vi "Swerve_Module Drive Config.vi"(5 "Max # Of Tries":i32, 6 "Send Cmd Timout(ms)":u32=300, 7 "Module Specific Data":T1, 8 "Error":errorcluster, 9 "Module Drive Config Data":T8={"ModuleDrive Ver"=0, "Output"={"Type"=enum."Counter-Clockwise", "Neutral"=enum."EEPROMSetting", "Max"={"FWD"=0.0, "REV"=0.0}, "Min"={"FWD"=0.0, "REV"=0.0}, "OL Ramp Rate (S)"=0.0, "Dead Band"=0.0}, "CL"={"Gains"={"P"=1.0, "I"=0.01, "D"=0.0, "F"=0.0}, "Error Allowed"={"High"=0.0, "Low"=0.0}, "I Zone"={"High"=10000.0, "Low"=-1000.0}, "Max Out"={"FWD"=1.0, "REV"=-1.0}, "Max I Accu"={"High"=10.0, "Low"=-10.0}, "CL Ramp Rate (S)"=0.0}, "VoltageComp"={"Enable"=FALSE, "Value"=0.0}} {"Output"."Min"."REV" format="%.2f"; "Output"."Min"."FWD" format="%.2f"; "Output"."Max"."REV" format="%.2f"; "Output"."Max"."FWD" format="%.2f"; "VoltageComp"."Value" format="%.1g"; "CL"."Max I Accu"."Low" format="%#.8f"; "CL"."Max I Accu"."High" format="%#.8f"; "CL"."Gains"."F" format="%#.8f"; "CL"."Gains"."D" format="%#.8f"; "CL"."Gains"."I" format="%#.8f"; "CL"."Gains"."P" format="%#.8f"; "CL"."Error Allowed"."Low" format="%#.8f"; "CL"."Error Allowed"."High" format="%#.8f"; "CL"."I Zone"."Low" format="%#.8f"; "CL"."I Zone"."High" format="%#.8f"; "CL"."Max Out"."REV" format="%.2f"; "CL"."Max Out"."FWD" format="%.2f"}, 11 "PhoenixMotorControlDevRef":T3={"DeviceStatus"={"status"=FALSE, "code"=0, "source"=""}, "Type"=enum."PWM", "PWM"={"PWM Channel"=enum."Invalid", "DeadBand"={"Name"="", "maxPositivePwm"=0, "minPositivePwm"=0, "centerPwm"=0, "maxNegativePwm"=0, "minNegativePwm"=0, "angularRange"=0}}, "CAN"={"Device Number"=0, "SetOutput VI Ref"=variant, "GetOutput VI Ref"=variant, "Enable VI Ref"=variant, "Disable VI Ref"=variant, "Data"=variant}, "Invert"=FALSE, "DIO PWM"={"PWM \"Enable\" Channel"=enum."Invalid", "DIOChannel"=enum."Invalid", "PWM Rate"=0.0}}) -> (0 "Error Out":errorcluster, 3 "PhoenixMotorControlDevRef Out Out":T3)   [LabVIEW 2023]
uses:
  <vilib>/Utility/Data Type/NI_Data Type.lvlib
  <vilib>/Rock Robotics/WPI/ThirdParty/Phoenix-LabVIEW/Motor Controller/Controls/CTRE_Phoenix_MotorControl_NeutralMode.ctl
  <vilib>/Rock Robotics/SystemInterfaces/DIO/FPGA_DIOPWMChannel.ctl
  <vilib>/Rock Robotics/WPI/PWM/WPI_PWMDeadband.ctl
  <vilib>/Rock Robotics/WPI/MotorControl/WPI_MotorControlType.ctl
  <vilib>/Rock Robotics/SystemInterfaces/DIO/FPGA_DIOChannel.ctl
  <vilib>/Rock Robotics/WPI/MotorControl/WPI_MotorControlDeviceRef.ctl
  Shared Code/TypeDefs/Cluster_High-Low.ctl
  Shared Code/TypeDefs/Cluster_PID Gains.ctl
  Shared Code/TypeDefs/Cluster_PID Config.ctl
  <vilib>/Rock Robotics/WPI/ThirdParty/Phoenix-LabVIEW/Motor Controller/Controls/CTRE_Phoenix_MotorControl_TalonFXInvertType.ctl
  Shared Code/TypeDefs/Cluster_Enable-Value DBL.ctl
  Shared Code/TypeDefs/Cluster_Swerve Module Drive Config Data.ctl
  Shared Code/TypeDefs/ENUM_Motor Index.ctl
  Shared Code/TypeDefs/Cluster_Module Specific Config Data.ctl
  Shared Code/TypeDefs/Cluster_FWD  REV Values.ctl
  Shared Code/TypeDefs/Cluster_Config Motor Output.ctl
panel:
  # "Tune to Output\nto 1023 Max"
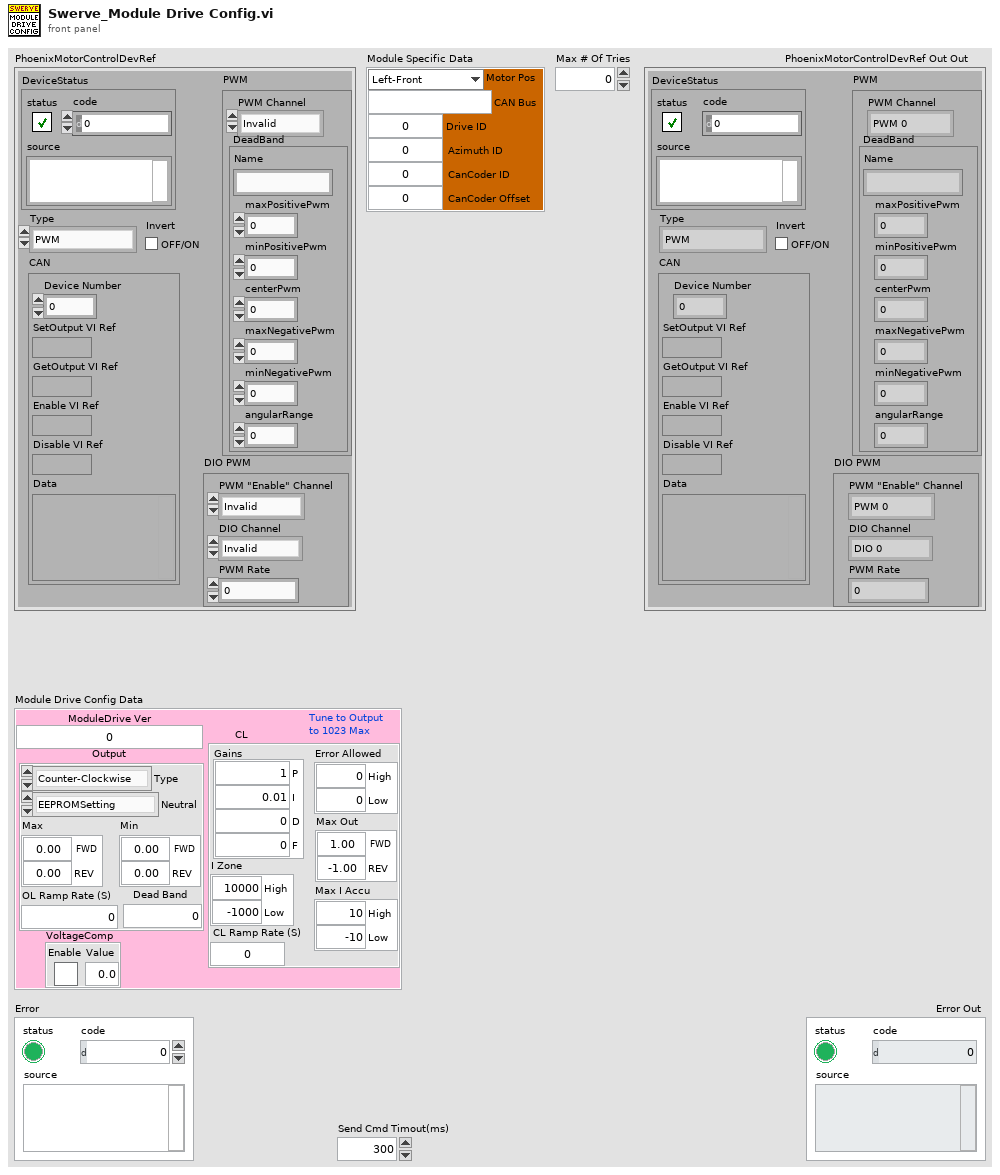
[diagram p1: front panel]
types:
  T1 = typedef "Cluster_Module Specific Config Data.ctl" = cluster{"Motor Pos":T2, "CAN Bus":string, "Drive ID":u8, "Azimuth ID":u8, "CanCoder ID":u8, "CanCoder Offset":dbl}
  T2 = typedef "ENUM_Motor Index.ctl" = enum16{"Left-Front", "Right-Front", "Left-Back", "Right-Back"}
  T3 = typedef "WPI_MotorControlDeviceRef.ctl" = cluster{"DeviceStatus":errorcluster, "Type":T4, "PWM":cluster{"PWM Channel":T5, "DeadBand":T6}, "CAN":cluster{"Device Number":u8, "SetOutput VI Ref":variant, "GetOutput VI Ref":variant, "Enable VI Ref":variant, "Disable VI Ref":variant, "Data":variant}, "Invert":bool, "DIO PWM":cluster{"PWM \"Enable\" Channel":T5, "DIOChannel":T7, "PWM Rate":dbl}}
  T4 = typedef "WPI_MotorControlType.ctl" = enum16{"PWM", "CAN", "DIO PWM"}
  T5 = typedef "FPGA_DIOPWMChannel.ctl" = enum8{"PWM 0", "PWM 1", "PWM 2", "PWM 3", "PWM 4", "PWM 5", "PWM 6", "PWM 7", "PWM 8", "PWM 9", "PWM MXP 0", "PWM MXP 1", "PWM MXP 2", "PWM MXP 3", "PWM MXP 4", "PWM MXP 5", "PWM MXP 6", "PWM MXP 7", "PWM MXP 8", "PWM MXP 9", "Invalid"}
  T6 = typedef "WPI_PWMDeadband.ctl" = cluster{"Name":string, "maxPositivePwm":i32, "minPositivePwm":i32, "centerPwm":i32, "maxNegativePwm":i32, "minNegativePwm":i32, "angularRange":u16}
  T7 = typedef "FPGA_DIOChannel.ctl" = enum8{"DIO 0", "DIO 1", "DIO 2", "DIO 3", "DIO 4", "DIO 5", "DIO 6", "DIO 7", "DIO 8", "DIO 9", "DIO MXP 0", "DIO MXP 1", "DIO MXP 2", "DIO MXP 3", "DIO MXP 4", "DIO MXP 5", "DIO MXP 6", "DIO MXP 7", "DIO MXP 8", "DIO MXP 9", "DIO MXP 10", "DIO MXP 11", "DIO MXP 12", "DIO MXP 13", "DIO MXP 14", "DIO MXP 15", "SPI Port CS1", "SPI Port CS2", "SPI Port CS3", "SPI Port MISO", "SPI Port MOSI", "Invalid"}
  T8 = typedef "Cluster_Swerve Module Drive Config Data.ctl" = cluster{"ModuleDrive Ver":u64, "Output":T9, "CL":T13, "VoltageComp":T16}
  T9 = typedef "Cluster_Config Motor Output.ctl" = cluster{"Type":T10, "Neutral":T11, "Max":T12, "Min":T12, "OL Ramp Rate (S)":dbl, "Dead Band":dbl}
  T10 = typedef "CTRE_Phoenix_MotorControl_TalonFXInvertType.ctl" = enum16{"Counter-Clockwise", "Clockwise"}
  T11 = typedef "CTRE_Phoenix_MotorControl_NeutralMode.ctl" = enum8{"EEPROMSetting", "Override to Coast", "Override to Brake"}
  T12 = typedef "Cluster_FWD  REV Values.ctl" = cluster{"FWD":dbl, "REV":dbl}
  T13 = typedef "Cluster_PID Config.ctl" = cluster{"Gains":T14, "Error Allowed":T15, "I Zone":T15, "Max Out":T12, "Max I Accu":T15, "CL Ramp Rate (S)":dbl}
  T14 = typedef "Cluster_PID Gains.ctl" = cluster{"P":dbl, "I":dbl, "D":dbl, "F":dbl}
  T15 = typedef "Cluster_High-Low.ctl" = cluster{"High":dbl, "Low":dbl}
  T16 = typedef "Cluster_Enable-Value DBL.ctl" = cluster{"Enable":bool, "Value":dbl}
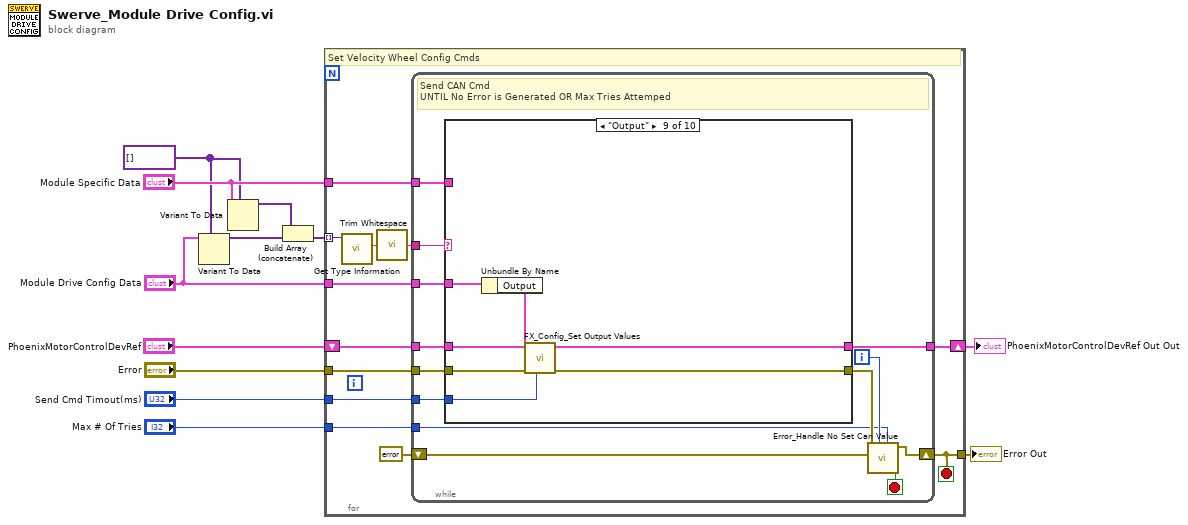
[diagram p0: block diagram]
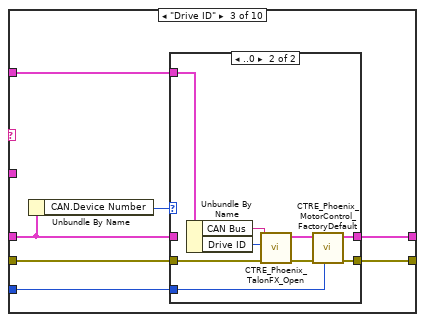
[diagram p4: hidden frame]
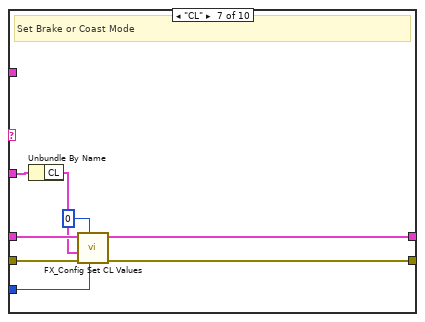
[diagram p9: hidden frame]
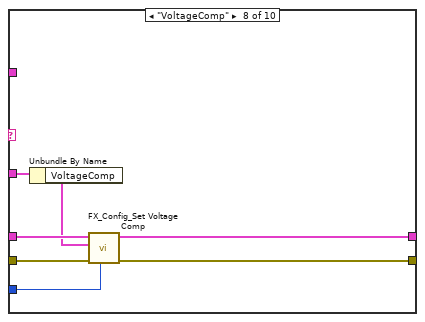
[diagram p10: hidden frame]
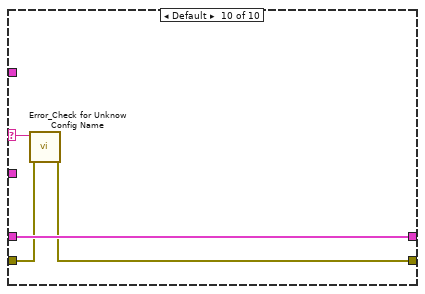
[diagram p11: hidden frame]
diagram:
  w4 = variant[] [] ("type")
  n1 = Variant To Data(type=w4, Variant="Module Drive Config Data") -> (data=w3:variant[])  [unwired: 1 in, 1 out]
  n2 = Variant To Data(type=w4, Variant="Module Specific Data") -> (data=w1:variant[])  [unwired: 1 in, 1 out]
  n3 = Build Array (concatenate)(w1, w3) -> (w2:variant[])
  n4 = for {
    tunnel: "Send Cmd Timout(ms)" -> [w23]
    shift-right: [w24] -> w9
    shift-left: "PhoenixMotorControlDevRef" -> [w21]
    tunnel: "Module Drive Config Data" -> [w22]
    tunnel: "Max # Of Tries" -> [w19]
    tunnel: w2 -> [w18] mode=indexing
    tunnel: "Error" -> [w20]
    tunnel: [w17] -> w8
    tunnel: "Module Specific Data" -> [w15]
    stop <- w17 stop-if-true
    # "Set Velocity Wheel Config Cmds"
    n5 = call <vilib>:"Get Type Information.vi"("variant"=w18) -> ("name"=w14:string)  [unwired: 6 in, 4 out]
    n6 = call <vilib>:"Trim Whitespace.vi"("string"=w14) -> ("trimmed string"=w13:string)  [unwired: 1 in]
    n7 = while {
      tunnel: [w29] -> w24
      tunnel: w23 -> [w35]
      shift-right: [w36] -> w17
      shift-left: errorcluster {"status"=FALSE, "code"=0, "source"=""} ("Error Out") -> [w34]
      tunnel: w20 -> [w32]
      tunnel: w21 -> [w31]
      tunnel: w22 -> [w30]
      tunnel: w19 -> [w28]
      tunnel: w13 -> [w27]
      tunnel: w15 -> [w25]
      i -> [w33]
      stop <- w26 stop-if-true
      # "Send CAN Cmd\nUNTIL No Error is Generated OR Max Tries Attemped"
      n8 = case shown="\"Output\"" w27 {
        selector: w27 -> [_ _ _ _ _ _ _ _ _ w91]
        tunnel: [w39 w41 w47 w61 w63 w65 w71 w80 w87 w89] -> w37
        tunnel: w35 -> [_ _ w45 _ _ _ w66 w74 w81 _]
        tunnel: w32 -> [w39 w41 w46 w61 w63 w65 w70 w79 w86 w88]
        tunnel: w31 -> [w38 w40 w43 w60 w62 w64 w73 w76 w83 w90]
        tunnel: w30 -> [_ _ _ _ _ _ w69 w77 w84 _]
        tunnel: [w38 w40 w42 w60 w62 w64 w72 w78 w85 w90] -> w29
        tunnel: w25 -> [_ _ w48 _ _ _ _ _ _ _]
        frame "Motor Pos" {
        }
        frame "CAN Bus" {
        }
        frame "Drive ID" {
          n9 = Unbundle By Name(w43) -> ("CAN.Device Number"=w44:u8)
          n10 = case shown="..0" w44 {
            tunnel: w48 -> [_ w56]
            tunnel: [w49 w55] -> w47
            tunnel: w46 -> [w49 w54]
            tunnel: w45 -> [_ w53]
            tunnel: w43 -> [w50 _]
            tunnel: [w50 w51] -> w42
            frame 1.. {
            }
            frame ..0 {
              n11 = Unbundle By Name(w56) -> ("CAN Bus"=w52:string, "Drive ID"=w57:u8)
              n12 = call <vilib>:"CTRE_Phoenix_TalonFX_Open.vi"("error in"=w54, "Device Number"=w57, "CAN Bus"=w52) -> ("error out"=w58:errorcluster, "PhoenixMotorControlDevRef"=w59:T3)  [unwired: 7 in]
              n13 = call <vilib>:"CTRE_Phoenix_MotorControl_FactoryDefault.vi"("timeoutMs"=w53, "error in"=w58, "PhoenixMotorControlDevRef"=w59) -> ("error out"=w55:errorcluster, "PhoenixMotorControlDevRef"=w51:T3)  [unwired: 7 in]
            }
          }
        }
        frame "Azimuth ID" {
        }
        frame "CanCoder ID" {
        }
        frame "CanCoder Offset" {
        }
        frame "CL" {
          # "Set Brake or Coast Mode"
          n14 = Unbundle By Name(w69) -> ("CL"=w68:T13)
          n15 = call "FX_Config Set CL Values.vi"("Send Cmd Timout(ms)"=w66, "SlotIdx"=0, "Error"=w70, "CL"=w68, "PhoenixMotorControlDevRef"=w73) -> ("Error Out"=w71:errorcluster, "PhoenixMotorControlDevRef Out"=w72:T3)  [unwired: 4 in, 1 out]
        }
        frame "VoltageComp" {
          n16 = Unbundle By Name(w77) -> ("VoltageComp"=w75:T16)
          n17 = call "FX_Config_Set Voltage Comp.vi"("Send Cmd Timout(ms)"=w74, "Error"=w79, "VoltageComp"=w75, "PhoenixMotorControlDevRef"=w76) -> ("Error Out"=w80:errorcluster, "PhoenixMotorControlDevRef Out"=w78:T3)  [unwired: 6 in]
        }
        frame "Output" {
          n18 = Unbundle By Name(w84) -> ("Output"=w82:T9)
          n19 = call "FX_Config_Set Output Values.vi"("Send Cmd Timout(ms)"=w81, "Error"=w86, "Output"=w82, "PhoenixMotorControlDevRef"=w83) -> ("Error Out"=w87:errorcluster, "PhoenixMotorControlDevRef Out"=w85:T3)  [unwired: 6 in]
        }
        frame Default {
          n20 = call "Error_Check for Unknow Config Name.vi"("error in (no error)"=w88, "Config Name"=w91) -> ("error out"=w89:errorcluster)  [unwired: 9 in]
        }
      }
      n21 = call "Error_Handle No Set Can Value.vi"("Max # Of Tries"=w28, "Loop Itteration"=w33, "Previous Error"=w34, "Error"=w37) -> ("Stop Out"=w26:bool, "Error Out"=w36:errorcluster)  [unwired: 6 in]
    }
  }
  "Error Out" <- w8
  "PhoenixMotorControlDevRef Out Out" <- w9
